vi "MCS_MoveRelative.vi"(1 "error in (no error)":errorcluster, 2 "Moving Distance (um)":dbl, 3 "Channel Index In":u32, 4 "System Index In":u32) -> (0 "error out":errorcluster)   [LabVIEW 2010]
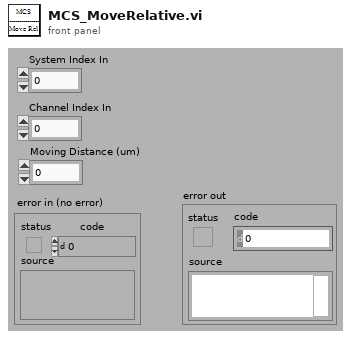
[diagram p1: front panel]
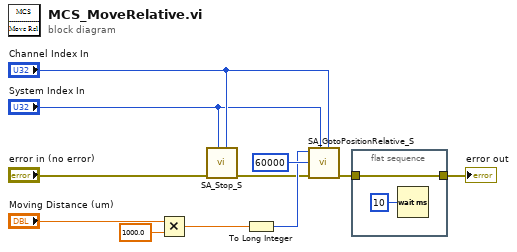
[diagram p0: block diagram]
diagram:
  n1 = Multiply(x="Moving Distance (um)", y=1000.0) -> (x*y=w8:dbl)
  n2 = call <vilib>:"SA_Stop_S.vi"("channelIndex"="Channel Index In", "systemIndex"="System Index In", "error in (no error)"="error in (no error)") -> ("error out"=w4:errorcluster)  [unwired: 8 in]
  n3 = To Long Integer(number=w8) -> (32bit integer=w6:i32)
  n4 = call <vilib>:"SA_GotoPositionRelative_S.vi"("channelIndex"="Channel Index In", "systemIndex"="System Index In", "error in (no error)"=w4, "holdTime"=u32 60000, "diff"=w6) -> ("error out"=w5:errorcluster)  [unwired: 6 in]
  n5 = flat-sequence {
    tunnel: w5 -> [w12]
    tunnel: [w12] -> w11
    frame #0 {
      n6 = Wait (ms)(milliseconds to wait=u32 10) -> ()  [unwired: 1 out]
    }
  }
  "error out" <- w11
